vi "main.vi"() -> ()   [LabVIEW 2021]
uses:
  NYPizzaStore/NYPizzaStore.lvclass
  ChicagoPizzaStore/ChicagoPizzaStore.lvclass
  Pizza/pizza types.ctl
  Pizza/Pizza.lvclass
panel:
  out "error out":errorcluster
  out "Messages":string
  # "Locals"
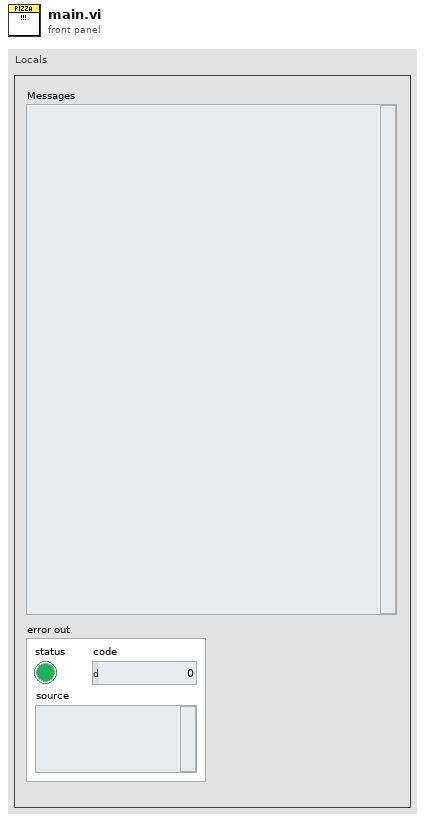
[diagram p1: front panel]
types:
  T1 = typedef "Pizza.lvclass/pizza types.ctl" = enum16{"Cheese", "Pepperoni"}
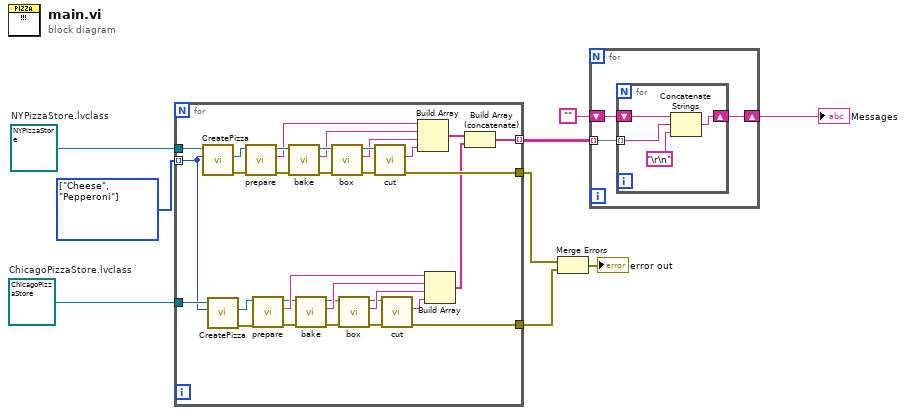
[diagram p0: block diagram]
diagram:
  w8 = T1[] [enum."Cheese", enum."Pepperoni"] items=["Cheese", "Pepperoni"] ("Pizza to order")
  w4 = refnum<class "ChicagoPizzaStore.lvclass"> refnum  # ChicagoPizzaStore.lvclass
  w9 = refnum<class "NYPizzaStore.lvclass"> refnum  # NYPizzaStore.lvclass
  n1 = for {
    tunnel: w9 -> [w41]
    tunnel: w8 -> [w25] mode=indexing
    tunnel: [w12] -> w7 mode=indexing
    tunnel: [w27] -> w3
    tunnel: w4 -> [w26]
    tunnel: [w10] -> w2
    n2 = call-dynamic "CreatePizza.vi"("Pizza to order"=w25, "NYPizzaStore in"=w41) -> ("error out"=w33:errorcluster, "Pizza object"=w40:refnum<class "Pizza.lvclass">)  [unwired: 7 in, 1 out]
    n3 = call-dynamic "CreatePizza.vi"("Pizza to order"=w25, "ChicagoPizzaStore in"=w26) -> ("error out"=w13:errorcluster, "Pizza object"=w14:refnum<class "Pizza.lvclass">)  [unwired: 7 in, 1 out]
    n4 = call "prepare.vi"("error in (no error)"=w33, "Pizza in"=w40) -> ("error out"=w38:errorcluster, "preparing message"=w32:string, "Pizza out"=w39:refnum<class "Pizza.lvclass">)  [unwired: 7 in]
    n5 = call "prepare.vi"("error in (no error)"=w13, "Pizza in"=w14) -> ("error out"=w16:errorcluster, "preparing message"=w21:string, "Pizza out"=w15:refnum<class "Pizza.lvclass">)  [unwired: 7 in]
    n6 = call "bake.vi"("error in (no error)"=w38, "Pizza in"=w39) -> ("error out"=w36:errorcluster, "baking message"=w31:string, "Pizza out"=w37:refnum<class "Pizza.lvclass">)  [unwired: 7 in]
    n7 = call "bake.vi"("error in (no error)"=w16, "Pizza in"=w15) -> ("error out"=w18:errorcluster, "baking message"=w22:string, "Pizza out"=w17:refnum<class "Pizza.lvclass">)  [unwired: 7 in]
    n8 = call "box.vi"("error in (no error)"=w36, "Pizza in"=w37) -> ("error out"=w34:errorcluster, "boxing message"=w30:string, "Pizza out"=w35:refnum<class "Pizza.lvclass">)  [unwired: 7 in]
    n9 = call "box.vi"("error in (no error)"=w18, "Pizza in"=w17) -> ("error out"=w20:errorcluster, "boxing message"=w23:string, "Pizza out"=w19:refnum<class "Pizza.lvclass">)  [unwired: 7 in]
    n10 = call "cut.vi"("error in (no error)"=w34, "Pizza in"=w35) -> ("error out"=w27:errorcluster, "baking message"=w29:string)  [unwired: 7 in, 1 out]
    n11 = call "cut.vi"("error in (no error)"=w20, "Pizza in"=w19) -> ("error out"=w10:errorcluster, "baking message"=w24:string)  [unwired: 7 in, 1 out]
    n12 = Build Array(w32, w31, w30, w29) -> (w28:string[])
    n13 = Build Array(w21, w22, w23, w24) -> (w11:string[])
    n14 = Build Array (concatenate)(w28, w11) -> (w12:string[])
  }
  n15 = Merge Errors(w3, w2) -> (→"error out":errorcluster)
  n16 = for {
    tunnel: w7 -> [w44] mode=indexing
    shift-right: [w42] -> w5
    shift-left: "" -> [w43]
    n17 = for {
      tunnel: w44 -> [w45] mode=indexing
      shift-right: [w47] -> w42
      shift-left: w43 -> [w48]
      n18 = Concatenate Strings(w48, w45, "\r\n") -> (w47:string)
    }
  }
  "Messages" <- w5
